vi "create logger string.vi"(1 "Event":string="Magnet initialized") -> (0 "Event Logger out":string)   [LabVIEW 2017]
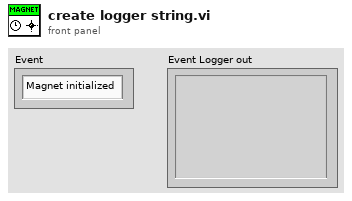
[diagram p1: front panel]
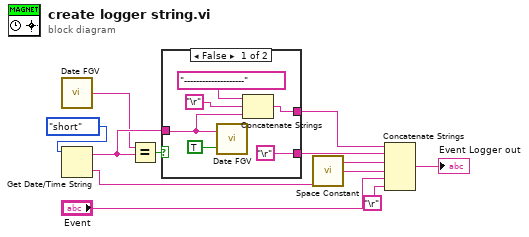
[diagram p0: block diagram]
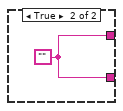
[diagram p2: hidden frame]
diagram:
  n1 = call "Date FGV.vi"() -> ("Date out"=w7:string)  [unwired: 2 in]
  n2 = Get Date/Time String(date format (0)=enum16{"short", "long", "abbreviated"}."short") -> (date string=w10:string, time string=w4:string)  [unwired: 2 in]
  n3 = Equal?(x=w7, y=w10) -> (x = y?=w9:bool)
  n4 = case shown="False" w9 {
    tunnel: [w15 w18] -> w2
    tunnel: w10 -> [w14 _]
    tunnel: ["\r" w18] -> w1
    frame False {
      n5 = call "Date FGV.vi"("Set?"=TRUE, "Date in"=w14) -> ()  [unwired: 1 out]
      n6 = Concatenate Strings("--------------------", "\r", w14) -> (w15:string)
    }
    frame True {
      w18 = ""
    }
  }
  n7 = call <vilib>:"Space Constant.vi"() -> ("String"=w3:string)
  n8 = Concatenate Strings(w2, w1, w4, w3, "Event", "\r") -> (→"Event Logger out":string)
